vi "GOOP_GetClassFolderFiles.vi"(11 "NewFolderPath":path) -> (3 "Array":path[](array[path]))   [LabVIEW 2020]
uses:
  <vilib>/Utility/lvfile.llb/NI_FileType.lvlib
  <vilib>/Utility/LVLibp/NI_PackedLibraryUtility.lvlib
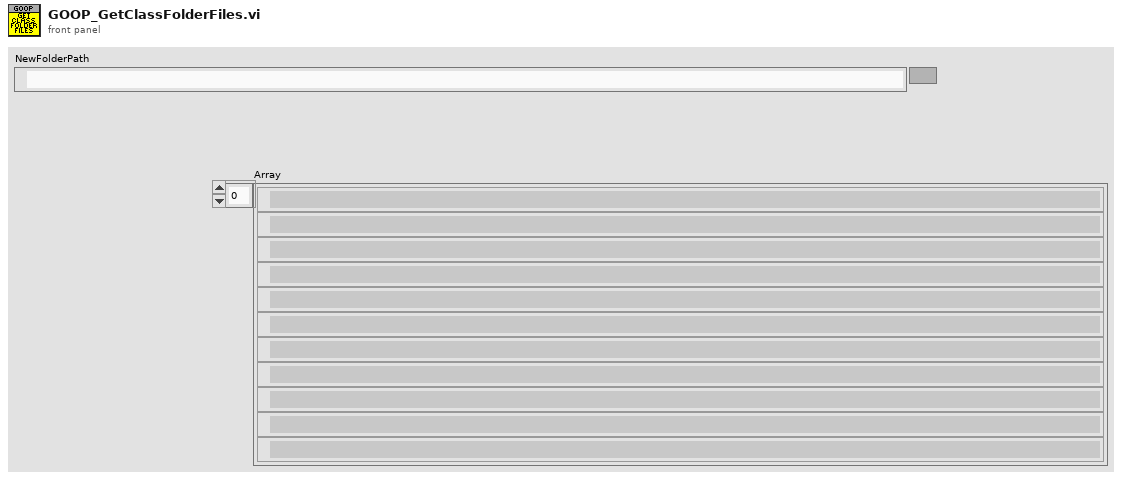
[diagram p1: front panel]
types:
  T1 = typedef "Librarian File List.ctl" = cluster{"name":string, "create date":u32, "mod date":u32, "type":string, "creator":string, "LV version":i32}[]
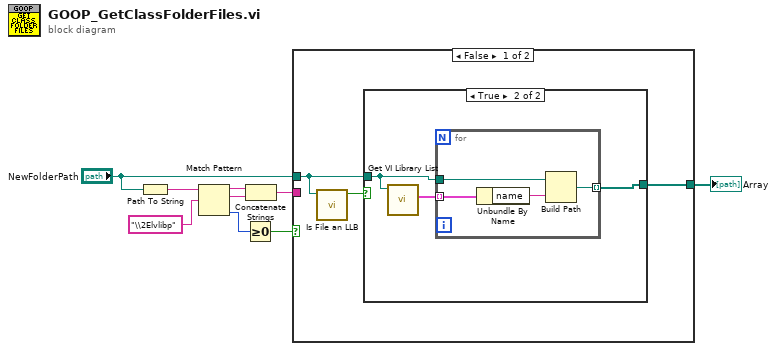
[diagram p0: block diagram]
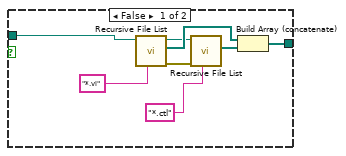
[diagram p2: hidden frame]
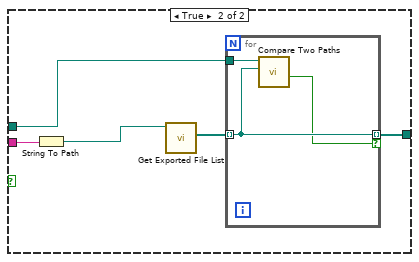
[diagram p3: hidden frame]
diagram:
  n1 = Path To String(path="NewFolderPath") -> (string=w8:string)
  n2 = Match Pattern(string=w8, regular expression="\\2Elvlibp") -> (before substring=w5:string, match substring=w4:string, offset past match=w6:i32)  [unwired: 1 in, 1 out]
  n3 = Greater Or Equal To 0?(x=w6) -> (x >= 0?=w2:bool)
  n4 = Concatenate Strings(w5, w4) -> (w1:string)
  n5 = case shown="False" w2 {
    tunnel: [w12 w28] -> w9
    tunnel: "NewFolderPath" -> [w10 w30]
    tunnel: w1 -> [_ w32]
    frame False {
      n6 = call <vilib>:"Is File an LLB.vi"("path"=w10) -> ("Is LLB?"=w11:bool)  [unwired: 9 in, 1 out]
      n7 = case shown="True" w11 {
        tunnel: [w20 w22] -> w12
        tunnel: w10 -> [w13 w21]
        frame False {
          n8 = call <vilib>:"Recursive File List.vi"("pattern"="*.vi", "Folder Path"=w13) -> ("error out"=w17:errorcluster, "All Files in Dir"=w18:path[], "dup Folder Path"=w15:path)  [unwired: 5 in, 2 out]
          n9 = call <vilib>:"Recursive File List.vi"("pattern"="*.ctl", "error in (no error)"=w17, "Folder Path"=w15) -> ("All Files in Dir"=w19:path[])  [unwired: 4 in, 4 out]
          n10 = Build Array (concatenate)(w18, w19) -> (w20:path[])
        }
        frame True {
          n11 = call <vilib>:"Get VI Library List.vi"("library path"=w21) -> ("file list"=w23:T1)  [unwired: 9 in, 1 out]
          n12 = for {
            tunnel: w23 -> [w27] mode=indexing
            tunnel: w21 -> [w25]
            tunnel: [w24] -> w22 mode=indexing
            n13 = Unbundle By Name(w27) -> ("name"=w26:string)
            n14 = Build Path(base path=w25, name or relative path=w26) -> (appended path=w24:path)
          }
        }
      }
    }
    frame True {
      n15 = String To Path(string=w32) -> (path=w31:path)
      n16 = call <vilib>:"Get Exported File List.vi"("packed library path"=w31) -> ("paths"=w29:path[])  [unwired: 8 in, 2 out]
      n17 = for {
        tunnel: w30 -> [w35]
        tunnel: w29 -> [w34] mode=indexing
        tunnel: [w34] -> w28 mode=indexing if=w33
        n18 = call <vilib>:"Compare Two Paths.vi"("Path 2"=w34, "Path 1"=w35) -> ("Path 2 Relative to Path 1?"=w33:bool)  [unwired: 6 in, 3 out]
      }
    }
  }
  "Array" <- w9
